vi "Memory.Pointer.External.Encapsulate.vi"(8 "error in (no error)":errorcluster, 10 "size":u64 format="%d bytes", 11 "address":u64 format="%016x") -> (0 "error out":errorcluster, 3 "external pointer":refnum<class "Memory.Pointer.External.lvclass">)   [LabVIEW 2016, in "Memory Manager.lvlib" / "Memory.Pointer.External.lvclass"]
doc: "Encapsulates an existing pointer allocated externally to LabVIEW to allow manipulation of that pointer using this library."
uses:
  Memory.Pointer.External.lvclass
  C:/Users/Ryan/Documents/Git/Sourcetree/LabVIEW-Memory-Manager/Source/Library/Classes/Pointer/Memory.Pointer.lvclass
  Pointer/Memory.Pointer.lvclass/Memory.Pointer.ctl
  Pointer/Memory.Pointer.lvclass
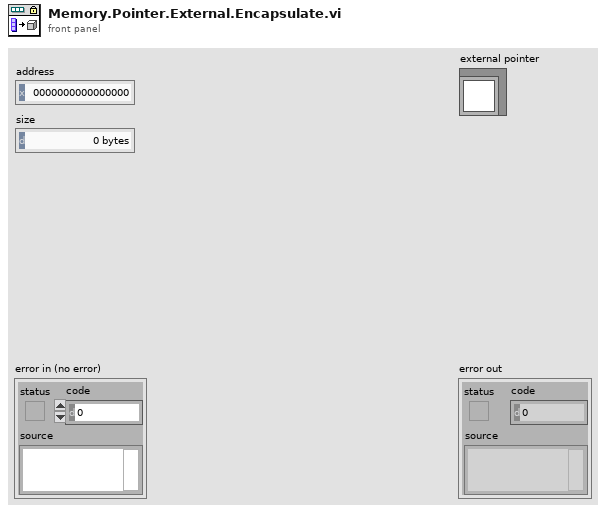
[diagram p1: front panel]
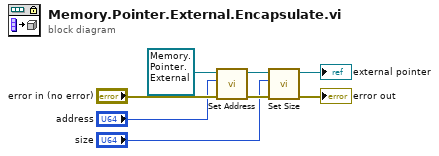
[diagram p0: block diagram]
diagram:
  n1 = call "Set Address.vi"("error in (no error)"="error in (no error)", "address"="address", "Pointer in"=refnum<class "Memory.Pointer.External.lvclass"> refnum ("pointer out")) -> ("error out"=w4:errorcluster, "Pointer out"=w6:refnum<class "Memory.Pointer.External.lvclass">)  [unwired: 7 in]
  n2 = call "Set Size.vi"("error in (no error)"=w4, "size"="size", "Pointer in"=w6) -> ("error out"=→"error out":errorcluster, "Pointer out"=→"external pointer":refnum<class "Memory.Pointer.External.lvclass">)  [unwired: 7 in]
